vi "1.vi"() -> ()   [LabVIEW 2017]
uses:
  <vilib>/Instr/_visa.llb/VISA Flush IO Buffer Mask.ctl
  <vilib>/Instr/_visa.llb/VISA Configure Serial Port (Instr).vi
panel:
  out "波形图表":u32(graph)
  in  "停止":bool
  out "读取缓冲区":string
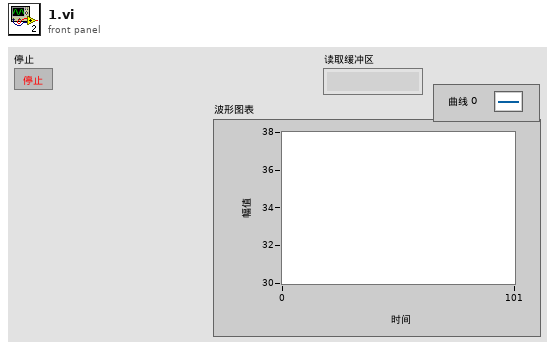
[diagram p1: front panel]
types:
  T1 = typedef "VISA Flush IO Buffer Mask.ctl" = u16
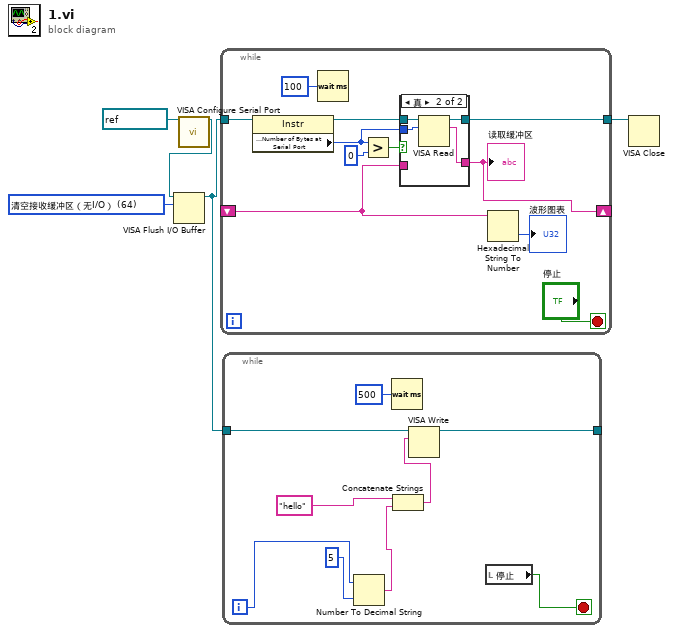
[diagram p0: block diagram]
diagram:
  w2 = T1 64 items=["清空接收缓冲区"=16, "向设备写入传输缓冲区"=32, "清空接收缓冲区（无I/O）"=64, "清空传输缓冲区"=128] ("Mask")
  n1 = call-poly "VISA Configure Serial Port"("VISA resource name"=refnum<visa-resource-name> "COM2") -> ("VISA resource name out"=w3:refnum<visa-resource-name>)  [unwired: 13 in, 1 out]
  n2 = VISA Flush I/O Buffer(VISA resource name=w3, mask (16)=w2) -> (VISA resource name out=w1:refnum<visa-resource-name>)  [unwired: 1 in, 1 out]
  n3 = while {
    tunnel: w1 -> [w14]
    tunnel: [w10] -> w4
    shift-right: [w8] -> _
    shift-left: _ -> [w7]
    stop <- "停止" stop-if-true
    n4 = property class="Instr"(reference=w14) -> (reference out=w11:refnum<visa-resource-name>, "Serial Settings:Number of Bytes at Serial Port"=w9:u32)  [unwired: 1 in, 1 out]
    n5 = Wait (ms)(milliseconds to wait=u32 100 ("等待时间（毫秒）")) -> ()  [unwired: 1 out]
    n6 = Greater?(x=w9, y=u32 0) -> (0:w12:bool)
    n7 = case shown="真" w12 {
      tunnel: w11 -> [w17 w22]
      tunnel: [w18 w21] -> w8
      tunnel: [w17 w20] -> w10
      tunnel: w7 -> [w18 _]
      tunnel: w9 -> [_ w19]
      frame False {
      }
      frame True {
        n8 = VISA Read(VISA resource name=w22, byte count=w19) -> (VISA resource name out=w20:refnum<visa-resource-name>, read buffer=w21:string)  [unwired: 1 in, 2 out]
      }
    }
    "读取缓冲区" <- w8
    n9 = Hexadecimal String To Number(string=w7) -> (number=→"波形图表":u32)  [unwired: 2 in, 1 out]
  }
  n10 = while {
    tunnel: w1 -> [w31]
    tunnel: [w27] -> _
    i -> [w25]
    stop <- w26 stop-if-true
    n11 = Number To Decimal String(number=w25, width (-)=i16 5 ("宽度(-)")) -> (decimal integer string=w23:string)
    n12 = Wait (ms)(milliseconds to wait=u32 500 ("等待时间（毫秒）")) -> ()  [unwired: 1 out]
    n13 = Concatenate Strings("hello" ("写入缓冲区"), w23) -> (w29:string)
    n14 = VISA Write(VISA resource name=w31, write buffer=w29) -> (VISA resource name out=w27:refnum<visa-resource-name>)  [unwired: 1 in, 2 out]
    n15 = local read "停止"() -> (w26:bool)
  }
  n16 = VISA Close(VISA resource name=w4) -> ()  [unwired: 1 in, 1 out]
